vi "CalcCubeDuration.vi"(8 "error in (no error)":errorcluster, 11 "Acquisition in":refnum<class "Acquisition.lvclass">) -> (0 "error out":errorcluster, 3 "Acquisition out":refnum<class "Acquisition.lvclass">)   [LabVIEW 2018, in "Acquisition.lvclass"]
uses:
  Acquisition.lvclass
  Acquisition.lvclass/Acquisition.ctl
  Interface/Interface.lvclass/Interface.ctl
  Channel/Channel.lvclass
  Interface/Interface.lvclass
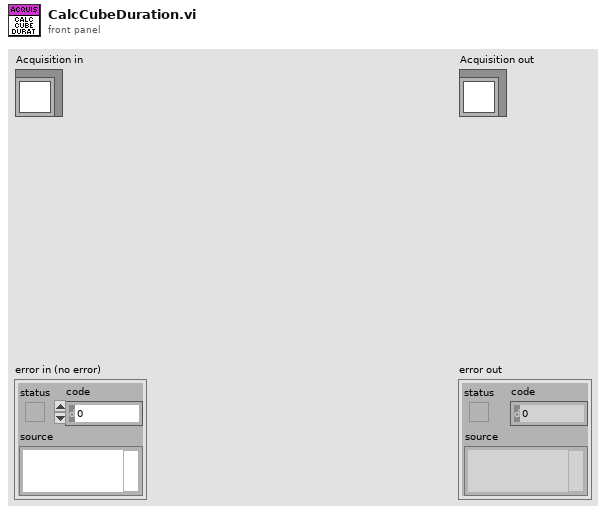
[diagram p1: front panel]
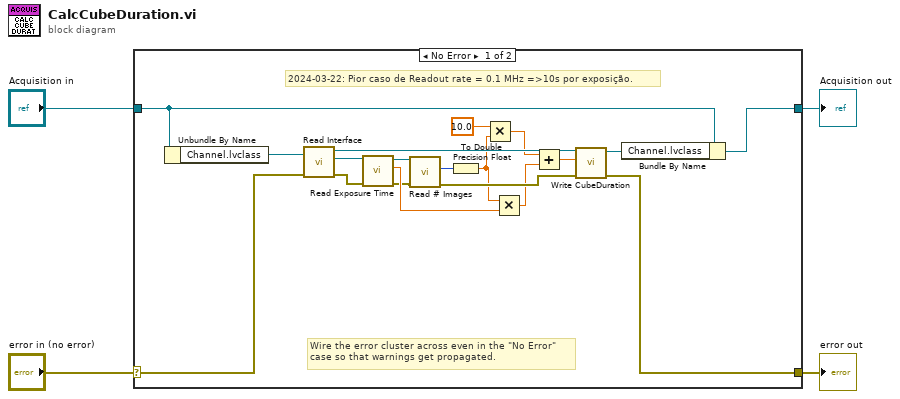
[diagram p0: block diagram]
diagram:
  n1 = case shown="No Error" "error in (no error)" {
    selector: "error in (no error)" -> [w14 w25]
    tunnel: [w10 w25] -> w3
    tunnel: [w15 w24] -> w1
    tunnel: "Acquisition in" -> [w17 w24]
    frame No Error {
      # "2024-03-22: Pior caso de Readout rate = 0.1 MHz =>10s por exposição."
      # "Wire the error cluster across even in the \"No Error\"\ncase so that warnings get propagated."
      n2 = Unbundle By Name(w17) -> ("Channel.lvclass"=w19:refnum<class "Channel.lvclass">)
      n3 = call-dynamic "Read Interface.vi"("error in (no error)"=w14, "Channel in"=w19) -> ("error out"=w13:errorcluster, "Interface.lvclass"=w21:refnum<class "Interface.lvclass">, "Channel out"=w18:refnum<class "Channel.lvclass">)  [unwired: 7 in]
      n4 = call "Read Exposure Time.vi"("error in (no error)"=w13, "Interface in"=w21) -> ("error out"=w12:errorcluster, "Exposure Time"=w22:dbl, "Interface out"=w20:refnum<class "Interface.lvclass">)  [unwired: 7 in]
      n5 = call-dynamic "Read # Images.vi"("error in (no error)"=w12, "Interface in"=w20) -> ("error out"=w11:errorcluster, "# Images"=w23:u32)  [unwired: 7 in, 1 out]
      n6 = To Double Precision Float(number=w23) -> (double precision float=w6:dbl)
      n7 = Multiply(x=10.0, y=w6) -> (x*y=w7:dbl)
      n8 = Multiply(x=w6, y=w22) -> (x*y=w8:dbl)
      n9 = Add(x=w7, y=w8) -> (x+y=w9:dbl)
      n10 = call-dynamic "Write CubeDuration.vi"("error in (no error)"=w11, "CubeDuration"=w9, "Channel in"=w18) -> ("error out"=w10:errorcluster, "Channel out"=w16:refnum<class "Channel.lvclass">)  [unwired: 7 in]
      n11 = Bundle By Name(cluster=w17, "Channel.lvclass"=w16) -> (w15:refnum<class "Acquisition.lvclass">)
    }
    frame Error {
    }
  }
  "error out" <- w3
  "Acquisition out" <- w1
